vi "solar_misc Export VIConPane Images.vi"() -> ()   [LabVIEW 2018]
doc: "This VI exports a folder of VIs connector pane images to the output directory."
panel:
  in  "Output Wiki Markup? (T)":bool=TRUE
  in  "OutputDir":path
  in  "Folders to Exclude":string[](array[string])=["_builds", "_dev", "_vipb", "_vip"]
  in  "error in (no error)":errorcluster
  out "error out":errorcluster
  out "Complete":dbl(slide) scale=0.0..100.0
  in  "RootDir":path=path "C:/Projects/solar/LV2016/solar"
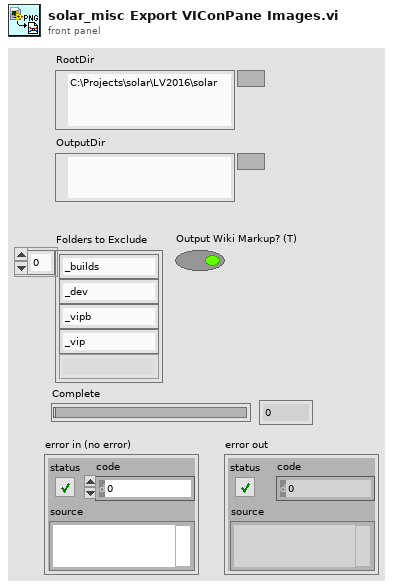
[diagram p1: front panel]
types:
  T1 = enum32{"invalid VI type", "Standard VI", "Control VI", "Global VI", "Polymorphic VI", "Configuration VI", "SubSystem", "Facade VI", "Method VI", "Statechart Diagram VI"}
  T2 = typedef "imagedata.ctl" = cluster{"image type":i32, "image depth":i32, "image":u8[], "mask":u8[], "colors":u32[], "Rectangle":cluster{"left":i16, "top":i16, "right":i16, "bottom":i16}}
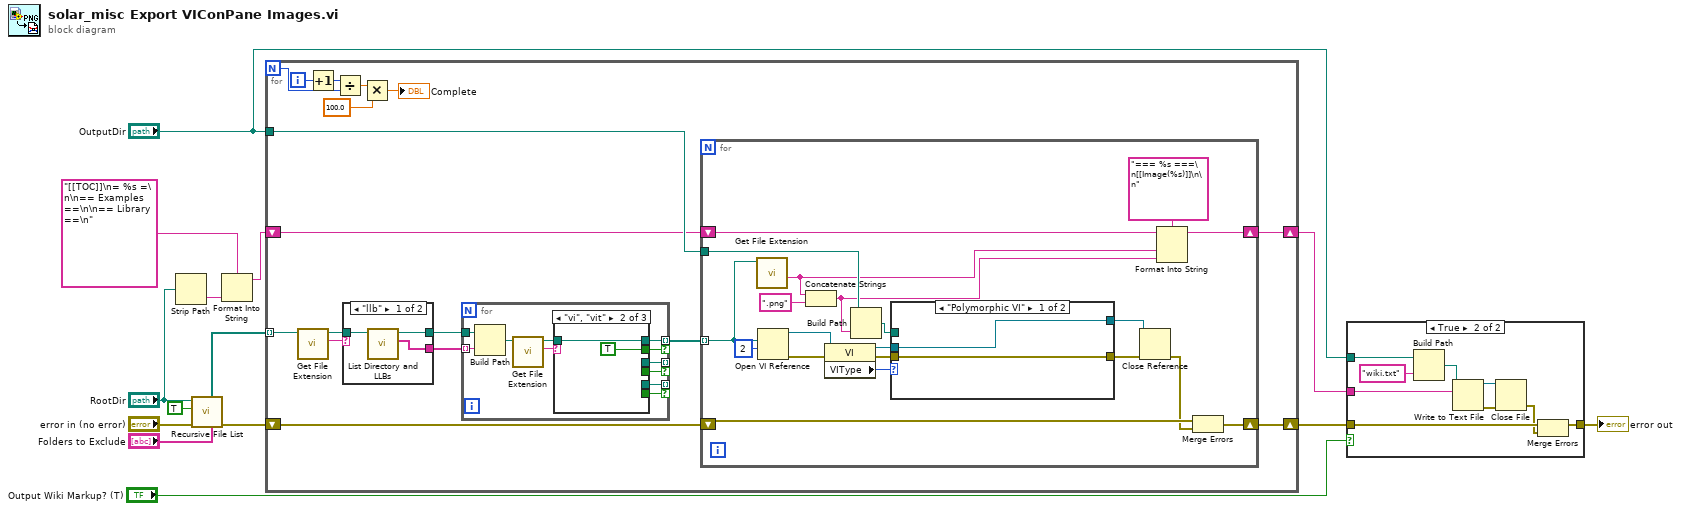
[diagram p0: block diagram]
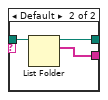
[diagram p3: hidden frame]
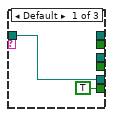
[diagram p4: hidden frame]
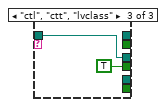
[diagram p5: hidden frame]
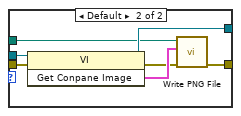
[diagram p6: hidden frame]
diagram:
  n1 = Strip Path(path="RootDir") -> (name=w7:string)  [unwired: 1 out]
  n2 = call <vilib>:"Recursive File List.vi"("Folders to Exclude"="Folders to Exclude", "error in (no error)"="error in (no error)", "Treat LLBs as Folders?"=TRUE, "Folder Path"="RootDir") -> ("error out"=w9:errorcluster, "All Folders"=w14:path[])  [unwired: 3 in, 3 out]
  n3 = Format Into String(format string="[[TOC]]\n= %s =\n\n== Examples ==\n\n== Library ==\n", w7) -> (resulting string=w5:string)  [unwired: 2 in, 1 out]
  n4 = for {
    N -> [w25]
    tunnel: w14 -> [w28] mode=indexing
    tunnel: "OutputDir" -> [w19]
    shift-right: [w18] -> w10
    shift-left: w9 -> [w17]
    shift-right: [w15] -> w3
    shift-left: w5 -> [w16]
    i -> [w26]
    n5 = call <vilib>:"Get File Extension.vi"("file"=w28) -> ("lowercase file extension"=w30:string, "dup file"=w29:path)  [unwired: 6 in, 3 out]
    n6 = Increment(x=w26) -> (x+1=w24:i32)
    n7 = Divide(x=w24, y=w25) -> (x/y=w23:dbl)
    n8 = case shown="\"llb\"" w30 {
      tunnel: w29 -> [w34 w37]
      tunnel: [w33 w36] -> w31
      tunnel: [w32 w35] -> w27
      frame "llb" {
        n9 = call <vilib>:"List Directory and LLBs.vi"("Folder Path"=w34) -> ("Files sans LLBs"=w32:string[], "dup Folder Path"=w33:path)  [unwired: 2 in, 7 out]
      }
      frame Default {
        n10 = List Folder(path=w37) -> (path out=w36:path, filenames=w35:string[])  [unwired: 3 in, 2 out]
      }
    }
    n11 = Multiply(x=w23, y=100.0) -> (x*y=→"Complete":dbl)
    n12 = for {
      tunnel: w31 -> [w48]
      tunnel: w27 -> [w47] mode=indexing
      tunnel: [w44] -> w20 mode=indexing if=w40
      tunnel: [w42] -> _ mode=indexing if=w41
      tunnel: [w39] -> _ mode=indexing if=w38
      n13 = Build Path(base path=w48, name or relative path=w47) -> (appended path=w46:path)
      n14 = call <vilib>:"Get File Extension.vi"("file"=w46) -> ("lowercase file extension"=w45:string, "dup file"=w43:path)  [unwired: 6 in, 3 out]
      n15 = case shown="\"vi\", \"vit\"" w45 {
        tunnel: [_ w52 _] -> w44
        tunnel: w43 -> [w50 w52 w53]
        tunnel: [_ _ w53] -> w42
        tunnel: [_ _ TRUE] -> w41
        tunnel: [_ TRUE _] -> w40
        tunnel: [w50 _ _] -> w39
        tunnel: [TRUE _ _] -> w38
        frame Default {
        }
        frame "vi", "vit" {
        }
        frame "ctl", "ctt", "lvclass" {
        }
      }
    }
    n16 = for {
      tunnel: w20 -> [w72] mode=indexing
      tunnel: w19 -> [w70]
      shift-right: [w69] -> w18
      shift-left: w17 -> [w68]
      shift-right: [w58] -> w15
      shift-left: w16 -> [w59]
      n17 = call <vilib>:"Get File Extension.vi"("file"=w72) -> ("filename without extension"=w56:string)  [unwired: 6 in, 4 out]
      n18 = Open VI Reference(vi path=w72, options=2) -> (vi reference=w64:refnum<vi>, error out=w74:errorcluster)  [unwired: 4 in]
      n19 = Concatenate Strings(w56, ".png" ("string")) -> (w55:string)
      n20 = property class="VI"(reference=w64, error in=w74) -> (reference out=w63:refnum<vi>, error out=w65:errorcluster, "VIType"=w60:T1)
      n21 = Build Path(base path=w70, name or relative path=w55) -> (appended path=w67:path)
      n22 = case shown="\"Polymorphic VI\"" w60 {
        tunnel: [w75 w83] -> w73
        tunnel: w67 -> [_ w81]
        tunnel: w65 -> [w76 w80]
        tunnel: w63 -> [w75 w79]
        tunnel: [w76 w77] -> w62
        frame "Polymorphic VI" {
        }
        frame Default {
          n23 = invoke class="VI" method="Get Conpane Image"(reference=w79, error in=w80) -> (reference out=w83:refnum<vi>, error out=w78:errorcluster, "Get Conpane Image"=w82:T2)  [unwired: 1 in]
          n24 = call <vilib>:"Write PNG File.vi"("error in (no error)"=w78, "image data"=w82, "path to PNG file"=w81) -> ("error out"=w77:errorcluster)  [unwired: 7 in, 1 out]
        }
      }
      n25 = Close Reference(reference=w73, error in (no error)=w62) -> (error out=w61:errorcluster)
      n26 = Format Into String(format string="=== %s ===\n[[Image(%s)]]\n\n", initial string=w59, w56, w55) -> (resulting string=w58:string)  [unwired: 1 in, 1 out]
      n27 = Merge Errors(w68, w61) -> (w69:errorcluster)
    }
  }
  n28 = case shown="True" "Output Wiki Markup? (T)" {
    tunnel: w10 -> [w84 w93]
    tunnel: "OutputDir" -> [_ w91]
    tunnel: w3 -> [_ w88]
    tunnel: [w84 w87] -> w2
    frame False {
    }
    frame True {
      n29 = Build Path(base path=w91, name or relative path="wiki.txt") -> (appended path=w89:path)
      n30 = Write to Text File(file (use dialog)=w89, text=w88) -> (refnum out=w85:refnum<file>, error out=w92:errorcluster)  [unwired: 2 in, 1 out]
      n31 = Close File(refnum=w85, error in=w92) -> (error out=w86:errorcluster)  [unwired: 1 out]
      n32 = Merge Errors(w93, w86) -> (w87:errorcluster)
    }
  }
  "error out" <- w2
